vi "BoxCollisionDetails.vi"(9 "direction in":cdb, 10 "position in":T1, 11 "class data in":refnum<class "BoundingBox.lvclass">) -> (3 "collisionAction out":T2)   [LabVIEW 2010, in "Labricks.lvlib" / "BoundingBox.lvclass"]
uses:
  BoundingBox.lvclass
  RenderBase/SceneObject_class/CollisionAction.ctl
  <vilib>/Utility/miscctls.llb/LV3DPointTypeDef.ctl
  BoundingBox.lvclass/BoundingBox.ctl
  RenderBase/SceneObject_class/SceneObject.lvclass
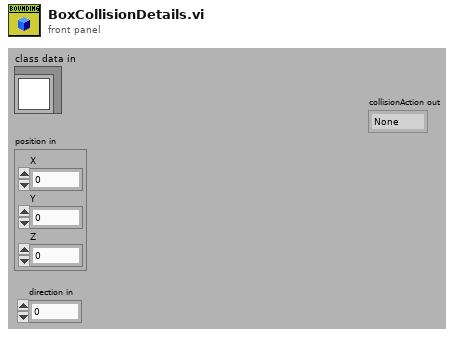
[diagram p1: front panel]
types:
  T1 = typedef "LV3DPointTypeDef.ctl" = cluster{"X":sgl, "Y":sgl, "Z":sgl}
  T2 = typedef "RenderBase.lvlib/SceneObject.lvclass/CollisionAction.ctl" = enum16{"None", "BounceX", "BounceY", "BounceXY"}
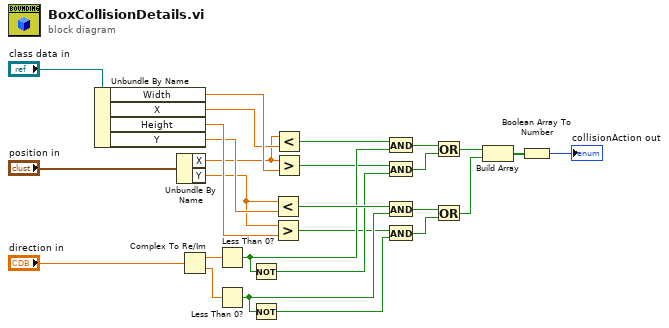
[diagram p0: block diagram]
diagram:
  n1 = Unbundle By Name("class data in") -> ("Width"=w22:sgl, "X"=w21:sgl, "Height"=w24:sgl, "Y"=w23:sgl)
  n2 = Unbundle By Name("position in") -> ("X"=w19:sgl, "Y"=w20:sgl)
  n3 = Complex To Re/Im(x + iy="direction in") -> (x=w26:dbl, y=w27:dbl)
  n4 = Less Than 0?(x=w26) -> (x < 0?=w13:bool)
  n5 = Less Than 0?(x=w27) -> (x < 0?=w10:bool)
  n6 = Not(x=w13) -> (.not. x?=w11:bool)
  n7 = Not(x=w10) -> (.not. x?=w9:bool)
  n8 = Less?(x=w20, y=w23) -> (x < y?=w16:bool)
  n9 = Greater?(x=w20, y=w24) -> (0:w8:bool)
  n10 = Less?(x=w19, y=w21) -> (x < y?=w14:bool)
  n11 = Greater?(x=w19, y=w22) -> (0:w12:bool)
  n12 = And(x=w14, y=w13) -> (x .and. y?=w7:bool)
  n13 = And(x=w12, y=w11) -> (x .and. y?=w6:bool)
  n14 = And(x=w16, y=w10) -> (x .and. y?=w4:bool)
  n15 = And(x=w8, y=w9) -> (x .and. y?=w5:bool)
  n16 = Or(x=w7, y=w6) -> (x .or. y?=w3:bool)
  n17 = Or(x=w4, y=w5) -> (x .or. y?=w2:bool)
  n18 = Build Array(w3, w2) -> (w1:bool[])
  n19 = Boolean Array To Number(Boolean array=w1) -> (number=→"collisionAction out":u32)
